vi "ELVIS III v1.0 DI Block Read Bank B.vi"(8 "error in (no error)":errorcluster, 9 "Number of Samples":u32=1000, 10 "Count (tick/s)":u32, 11 "DI Block Channels FPGA Reference":T1) -> (0 "error out":errorcluster, 3 "Data by Channel":bool[][](array[boolean]))   [LabVIEW 2021]
uses:
  <vilib>/myRIO/Common/Instrument Driver Framework/ELVIS III v1.0/DI Block/typedefs/ELVIS III DI Block FPGA Reference.ctl
  <vilib>/Utility/error.llb/Error Cluster From Error Code.vi
  <vilib>/rvi/errors/niLvFpgaAdjustHostInterfaceError.vi
  <vilib>/rvi/interface/nirviMethod/nirviMethod.xnode
  <vilib>/rvi/interface/nirviReadWriteControl/nirviReadWriteControl.xnode
  <vilib>/rvi/interface/Simulation/niFpgaSimulationCallBeginRW.vi
  <vilib>/rvi/errors/niLvFpgaMergeErrorWithErrorCode.vi
  NiFpgaLv.dll
  <vilib>/FPGAPlugInAG/Dynamic/niLvFpga_ReadFifo_Dynamic.vi
  <vilib>/FPGAPlugInAG/Dynamic/niLvFpga_StartFifo_Dynamic.vi
  <vilib>/FPGAPlugInAG/Dynamic/niLvFpga_StopFifo_Dynamic.vi
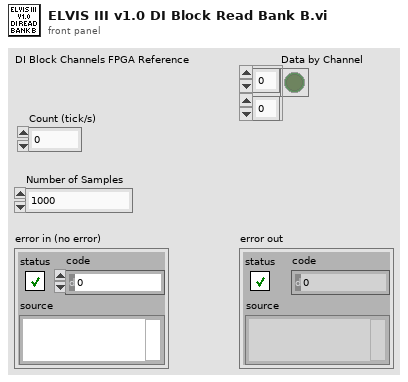
[diagram p1: front panel]
types:
  T1 = typedef "ELVIS III DI Block FPGA Reference.ctl" = refnum<k20>
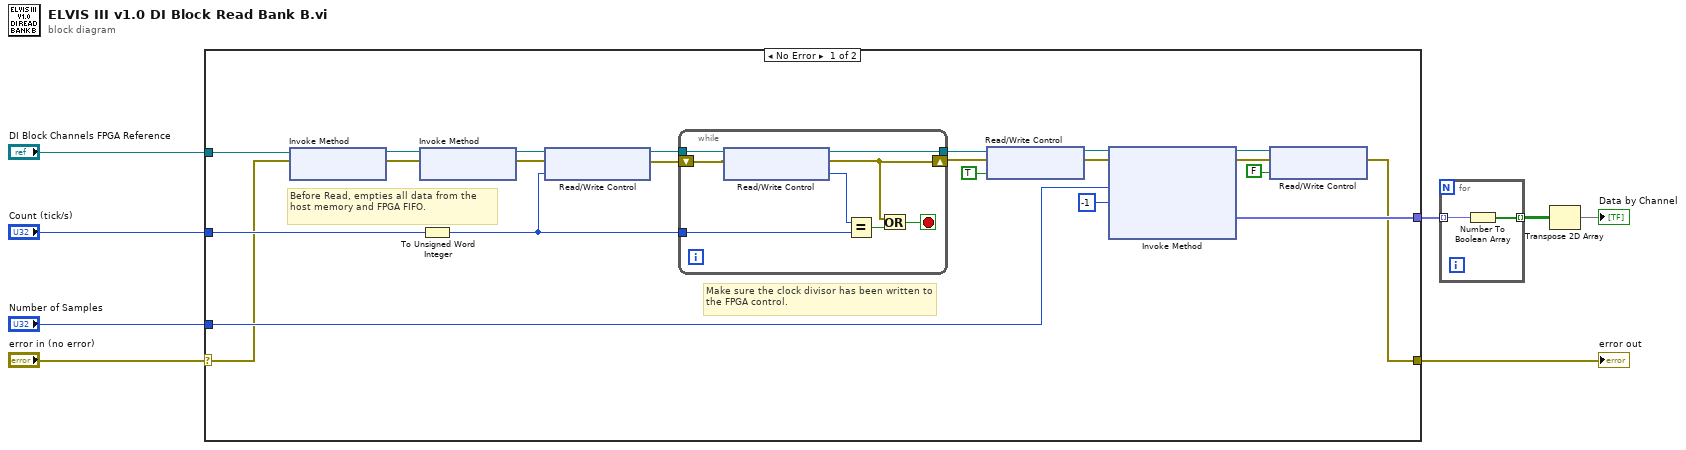
[diagram p0: block diagram]
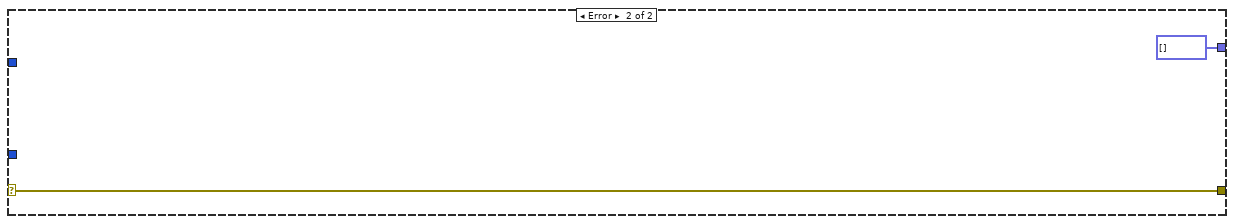
[diagram p2: hidden frame]
diagram:
  n1 = case shown="No Error" "error in (no error)" {
    selector: "error in (no error)" -> [w25 w40]
    tunnel: [w27 w40] -> w7
    tunnel: "Number of Samples" -> [w29 _]
    tunnel: "DI Block Channels FPGA Reference" -> [w30 _]
    tunnel: [w28 fxp<+,20,20>[] [] ("Data")] -> w4
    tunnel: "Count (tick/s)" -> [w26 _]
    frame No Error {
      # "Make sure the clock divisor has been written to the FPGA control."
      # "Before Read, empties all data from the host memory and FPGA FIFO."
      n2 = xnode "Invoke Method"("FPGA VI Reference In"=w30, "error in"=w25) -> ("FPGA VI Reference Out"=w24:T1, "error out"=w23:errorcluster)
      n3 = xnode "Invoke Method"("FPGA VI Reference In"=w24, "error in"=w23) -> ("FPGA VI Reference Out"=w22:T1, "error out"=w21:errorcluster)
      n4 = To Unsigned Word Integer(number=w26) -> (unsigned 16bit integer=w9:u16)
      n5 = xnode "Read/Write Control"("FPGA VI Reference In"=w22, "error in"=w21, "DI.B.DMA_CNTR"=w9) -> ("FPGA VI Reference Out"=w13:T1, "error out"=w12:errorcluster)
      n6 = while {
        tunnel: w13 -> [w35]
        tunnel: [w34] -> w11
        shift-right: [w33] -> w10
        shift-left: w12 -> [w32]
        tunnel: w9 -> [w38]
        stop <- w36 stop-if-true
        n7 = xnode "Read/Write Control"("FPGA VI Reference In"=w35, "error in"=w32) -> ("FPGA VI Reference Out"=w34:T1, "error out"=w33:errorcluster, "DI.B.DMA_CNTR"=w31:u16)
        n8 = Equal?(x=w31, y=w38) -> (x = y?=w37:bool)
        n9 = Or(x=w33, y=w37) -> (x .or. y?=w36:bool)
      }
      n10 = xnode "Read/Write Control"("FPGA VI Reference In"=w11, "error in"=w10, "DI.B.DMA_ENA"=TRUE ("Flag_DI")) -> ("FPGA VI Reference Out"=w19:T1, "error out"=w18:errorcluster)
      n11 = xnode "Invoke Method"("FPGA VI Reference In"=w19, "error in"=w18, "Number of Elements"=w29, "Timeout (ms)"=-1) -> ("FPGA VI Reference Out"=w16:T1, "error out"=w15:errorcluster, "Data"=w28:fxp<+,20,20>[])  [unwired: 1 out]
      n12 = xnode "Read/Write Control"("FPGA VI Reference In"=w16, "error in"=w15, "DI.B.DMA_ENA"=FALSE ("Flag")) -> ("error out"=w27:errorcluster)  [unwired: 1 out]
    }
    frame Error {
    }
  }
  "error out" <- w7
  n13 = for {
    tunnel: w4 -> [w42] mode=indexing
    tunnel: [w41] -> w2 mode=indexing
    n14 = Number To Boolean Array(number=w42) -> (Boolean array=w41:bool[])
  }
  n15 = Transpose 2D Array(2D array=w2) -> (transposed array=→"Data by Channel":bool[][])
